vi "Get Tag Name List.vi"(7 "chan prop table":string[][](array[string])) -> (8 "list of tags":string[](array[string]))   [LabVIEW 2010]
doc: "Extracts the column of Tag Names (col.1) from the input Channel Properties Table. Nothing more than a simple index array function."
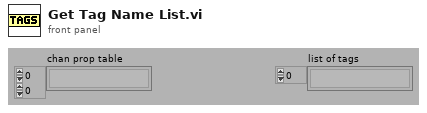
[diagram p1: front panel]
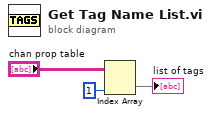
[diagram p0: block diagram]
diagram:
  n1 = Index Array(array="chan prop table", index (col)=1 ("disabled index (col)")) -> (element=→"list of tags":string[])  [unwired: 1 in]
